vi "SolveIntersectionLine.vi"(6 "P (cm)":cluster{"x":dbl, "y":dbl, "z":dbl}={"x"=1.0, "y"=-5.0, "z"=1.0} {"x" format="%.2f"; "z" format="%.2f"; "y" format="%.2f"}, 7 "P Variables":T1 {"Dtemp" format="%.2f"; "B" format="%.2f"; "A" format="%.2f"; "thetaw" format="%.2f"; "phih" format="%.2f"; "r (cm)" format="%.2f"}, 8 "min":dbl format="%.2f", 9 "max":dbl format="%.2f", 10 "strip":cluster{"radius":dbl, "h":dbl, "a":dbl}={"radius"=10.0, "h"=5.0, "a"=4.0} {"radius" format="%.2f"; "a" format="%.2f"; "h" format="%.2f"}, 11 "Variables":T2={"sound spd (cm/s)"=150000, "time step (s)"=1e-09} {"time step (s)" format="%.2e"}) -> (0 "rmin":dbl format="%.2f", 1 "slice thetas":dbl[][](array[numeric]) format="%.4f", 2 "sigma":dbl[](array[numeric]) format="%.2f", 3 "d":dbl[](array[numeric]) format="%.2f", 4 "wedge delay pts":i32)   [LabVIEW 2022 SP3]
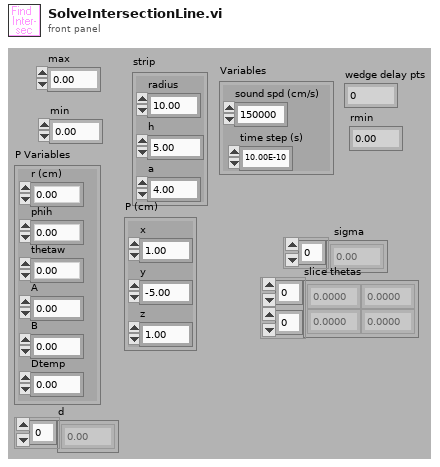
[diagram p1: front panel]
types:
  T1 = cluster{"r (cm)":dbl, "phih":dbl, "thetaw":dbl, "A":dbl, "B":dbl, "Dtemp":dbl}
  T2 = cluster{"sound spd (cm/s)":i32, "time step (s)":sgl}
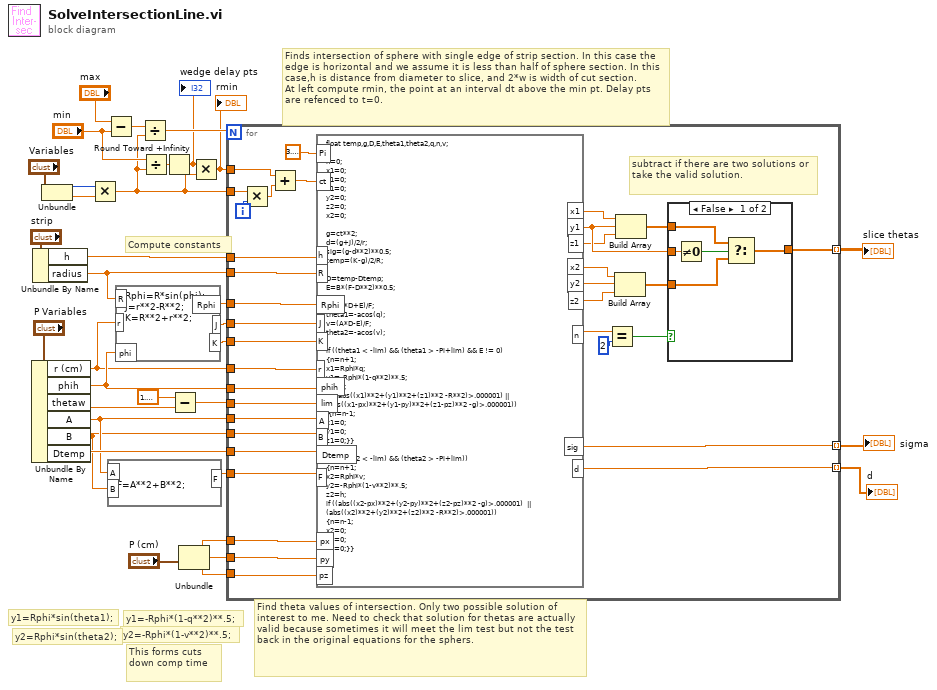
[diagram p0: block diagram]
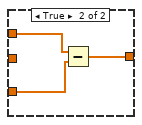
[diagram p2: hidden frame]
diagram:
  # "This forms cuts down comp time"
  # "y2=Rphi*sin(theta2);"
  # "y1=Rphi*sin(theta1);"
  # "y2=-Rphi*(1-v**2)**.5;"
  # "y1=-Rphi*(1-q**2)**.5;"
  # "Compute constants"
  # "Find theta values of intersection. Only two possible solution of interest to me. Need to check that solution for thetas are actually valid because sometimes it will meet the lim test but not the test back in the original equations for the sphers."
  # "Finds intersection of sphere with single edge of strip section. In this case the edge is horizontal and we assume it is less than half of sphere section. In this case,h is distance from diameter to slice, and 2*w is width of cut section.\nAt left compute rmin, the point at an interval dt above the min pt. Delay pts are refenced to t=0."
  n1 = Unbundle By Name("P Variables") -> ("r (cm)"=w6:dbl, "phih"=w25:dbl, "thetaw"=w16:dbl, "A"=w4:dbl, "B"=w3:dbl, "Dtemp"=w27:dbl)
  n2 = Unbundle By Name("strip") -> ("h"=w23:dbl, "radius"=w9:dbl)
  n3 = Unbundle("Variables") -> ("sound spd (cm/s)"=w29:i32, "time step (s)"=w28:sgl)
  n4 = Multiply(x=w29, y=w28) -> (x*y=w19:sgl)
  n5 = Subtract(x="max", y="min") -> (x-y=w33:dbl)
  n6 = formula code="F=A**2+B**2;"("A"=w4, "B"=w3) -> ("F"=w5:dbl)
  n7 = formula code="Rphi=R*sin(phi);\nJ=r**2-R**2;\nK=R**2+r**2;"("R"=w9, "phi"=w25, "r"=w6) -> ("Rphi"=w24:dbl, "J"=w7:dbl, "K"=w8:dbl)
  n8 = Divide(x=w33, y=w19) -> (x/y=w31:dbl)
  n9 = Divide(x="min", y=w19) -> (x/y=w20:dbl)
  n10 = Round Toward +Infinity(x=w20) -> (ceil(x): smallest int >= x=w17:dbl)
  "wedge delay pts" <- w17
  n11 = Subtract(x=1.5707963267948966, y=w16) -> (x-y=w14:dbl)
  n12 = Unbundle("P (cm)") -> ("x"=w12:dbl, "y"=w11:dbl, "z"=w10:dbl)
  n13 = Multiply(x=w17, y=w19) -> (x*y=w18:dbl)
  "rmin" <- w18
  n14 = for {
    N: w31 -> [_]
    tunnel: w9 -> [w56]
    tunnel: w19 -> [w68]
    tunnel: w6 -> [w64]
    tunnel: w27 -> [w63]
    tunnel: w3 -> [w62]
    tunnel: w4 -> [w61]
    tunnel: w14 -> [w60]
    tunnel: w25 -> [w59]
    tunnel: w24 -> [w58]
    tunnel: w23 -> [w57]
    tunnel: [w45] -> w22 mode=indexing
    tunnel: w18 -> [w52]
    tunnel: w12 -> [w51]
    tunnel: w11 -> [w50]
    tunnel: w10 -> [w49]
    tunnel: w5 -> [w48]
    tunnel: w8 -> [w47]
    tunnel: w7 -> [w46]
    tunnel: [w36] -> w2 mode=indexing
    tunnel: [w35] -> w1 mode=indexing
    i -> [w67]
    # "subtract if there are two solutions or take the valid solution."
    n15 = Multiply(x=w68, y=w67) -> (x*y=w69:sgl)
    n16 = Add(x=w52, y=w69) -> (x+y=w65:dbl)
    n17 = formula code="float temp,g,D,E,theta1,theta2,q,n,v;\n\nn=0;\nx1=0;\ny1=0;\nz1=0;\ny2=0;\nz2=0;\nx2=0;\n\ng=ct**2;\nd=(g+J)/2/r;\nsig=(g-d**2)**0.5;\ntemp=(K-g)/2/R;\n\nD=temp-Dtemp;\nE=B*(F-D**2)**0.5;\n\nq=(A*D+E)/F;\ntheta1=-acos(q);\nv=(A*D-E)/F;\ntheta2=-acos(v);\n\nif ((theta1 < -lim) && (theta1 > -Pi+lim) && E != 0)\n{n=n+1;\nx1=Rphi*q;\ny1=-Rphi*(1-q**2)**.5;\nz1=h;\nif ((abs((x1)**2+(y1)**2+(z1)**2 -R**2)>.000001) || (abs((x1-px)**2+(y1-py)**2+(z1-pz)**2 -g)>.000001))\n {n=n-1;\nx1=0;\ny1=0;\nz1=0;}}\n\nif ((theta2 < -lim) && (theta2 > -Pi+lim))\n{n=n+1;\nx2=Rphi*v;\ny2=-Rphi*(1-v**2)**.5;\nz2=h;\nif ((abs((x2-px)**2+(y2-py)**2+(z2-pz)**2 -g)>.000001)  || (abs((x2)**2+(y2)**2+(z2)**2 -R**2)>.000001))\n{n=n-1;\nx2=0;\ny2=0;\nz2=0;}}"("ct"=w65, "R"=w56, "Pi"=3.141592653589793, "r"=w64, "phih"=w59, "lim"=w60, "A"=w61, "B"=w62, "Dtemp"=w63, "Rphi"=w58, "h"=w57, "px"=w51, "py"=w50, "pz"=w49, "F"=w48, "J"=w46, "K"=w47) -> ("d"=w35:dbl, "sig"=w36:dbl, "x1"=w42:dbl, "y1"=w41:dbl, "z1"=w40:dbl, "x2"=w39:dbl, "y2"=w38:dbl, "z2"=w37:dbl, "n"=w43:dbl)
    n18 = Equal?(x=w43, y=2) -> (x = y?=w44:bool)
    n19 = Build Array(w39, w38, w37) -> (w53:dbl[])
    n20 = Build Array(w42, w41, w40) -> (w54:dbl[])
    n21 = case shown="False" w44 {
      tunnel: w54 -> [w72 w77]
      tunnel: w53 -> [w73 w76]
      tunnel: [w71 w75] -> w45
      tunnel: w41 -> [w70 _]
      frame False {
        n22 = Not Equal To 0?(x=w70) -> (x != 0?=w74:bool)
        n23 = Select(t=w72, s=w74, f=w73) -> (s? t:f=w71:dbl[])
      }
      frame True {
        n24 = Subtract(x=w77, y=w76) -> (x-y=w75:dbl[])
      }
    }
  }
  "sigma" <- w2
  "slice thetas" <- w22
  "d" <- w1
